vi "Time Estimate.vi"(8 "error in (no error)":errorcluster, 9 "expmode":i32, 10 "scantype":T1(ring), 11 "Magna Power Scan.lvclass":refnum<class "Magna Current Scan.lvclass">) -> (0 "error out":errorcluster, 1 "Time Estimate":string, 2 "time":dbl[unit], 3 "Magna Power Scan.lvclass out":refnum<class "Magna Current Scan.lvclass">)   [LabVIEW 2012, in "Magna Current Scan.lvclass"]
doc: "(Dynamic) Return an estimate of the time remaining to scan over this Scanner's preconfigured Range."
uses:
  Magna Current Scan.lvclass
  Magna Current Scan.lvclass/Magna Current Scan.ctl
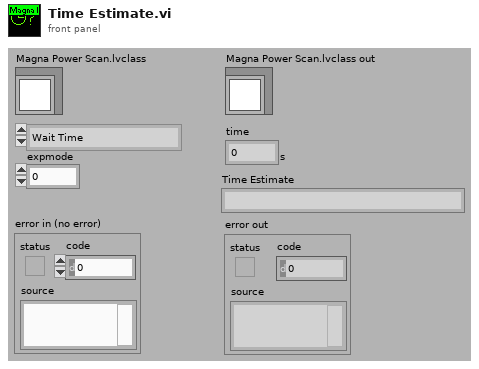
[diagram p1: front panel]
types:
  T1 = enum16{"Wait Time", "Pulse Width", "Wavelength", "Magnetic Field", "rf Scan"}
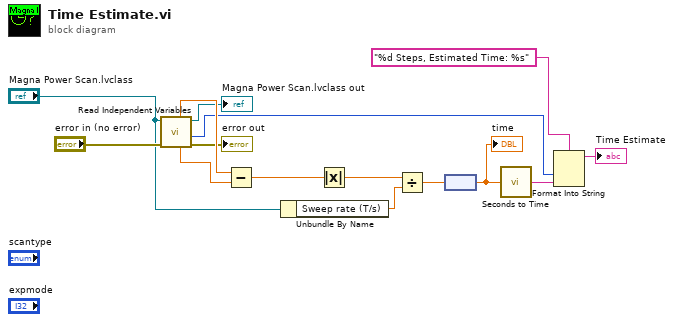
[diagram p0: block diagram]
diagram:
  n1 = call-dynamic "Read Independent Variables.vi"("error in (no error)"="error in (no error)", "Scanner.lvclass in"="Magna Power Scan.lvclass") -> ("error out"=→"error out":errorcluster, "size"=w6:i32, "Scanner.lvclass out"=→"Magna Power Scan.lvclass out":refnum<class "Magna Current Scan.lvclass">, "min value"=w9:dbl, "max value"=w10:dbl)  [unwired: 4 in, 1 out]
  n2 = Subtract(x=w10, y=w9) -> (x-y=w15:dbl)
  n3 = Unbundle By Name("Magna Power Scan.lvclass") -> ("Sweep rate (T/s)"=w13:dbl)
  n4 = Absolute Value(x=w15) -> (abs(x)=w14:dbl)
  n5 = Divide(x=w14, y=w13) -> (x/y=w5:dbl)
  n6 = node(w5) -> (w3:dbl[unit])
  "time" <- w3
  n7 = call "Seconds to Time.vi"("Seconds"=w3) -> ("Time"=w8:string)
  n8 = Format Into String(format string="%d Steps, Estimated Time: %s", w6, w8) -> (resulting string=→"Time Estimate":string)  [unwired: 2 in, 1 out]
